vi "Measure.vi"(5 "Progress Ref":refnum<vi>, 7 "XY Graph Reference":refnum<vi>, 8 "error in (no error)":errorcluster, 11 "MCCW ACLR in":refnum<class "MCCW ACLR.lvclass">) -> (0 "error out":errorcluster, 2 "Results":T1[](array[typedef]), 3 "MCCW ACLR out":refnum<class "MCCW ACLR.lvclass">)   [LabVIEW 2020, in "MCCW ACLR.lvclass"]
uses:
  MCCW ACLR.lvclass
  C:/Sandbox/RF Bench/Source Code/WiSpry Test Framework/Measurements/Measurement.lvclass
  XML Handler/Controls/Result Cluster.ctl
  Path Control/Paths.ctl
  MCCW ACLR.lvclass/MCCW ACLR.ctl
  Measurement.lvclass/Measurement.ctl
  Instruments/Spectrum Analyzer/Spectrum Analyzer.lvclass/Spectrum Analyzer.ctl
  Instruments/Vector Signal Generator/Vector Signal Generator.lvclass
  Instruments/Spectrum Analyzer/Spectrum Analyzer.lvclass
  Measurement.lvclass
  Path Control/PathControl.lvclass
  XML Handler/XML Handler.lvclass
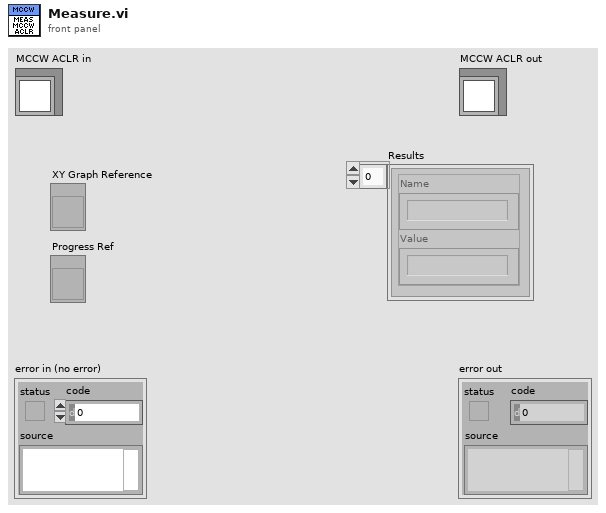
[diagram p1: front panel]
types:
  T1 = typedef "XML Handler.lvclass/Result Cluster.ctl" = cluster{"Name":string, "Value":string}
  T2 = typedef "PathControl.lvclass/Paths.ctl" = enum16{"SigGen 1 -> DUT", "SigGen 2 -> DUT", "SigGen 1 -> PM 1", "SigGen 1 -> PM 2", "DUT -> SA", "DUT -> PM 2", "VSG -> DUT", "SigGen 2 -> PM 1", "SigGen 2 -> PM 2"}
  T3 = cluster{"List":dbl[], "Index":i32, "Last":bool, "BW [MHz]":dbl}
  T4 = cluster{"Number of Measurements":u32, "Current Measurement":u32, "Last":bool}
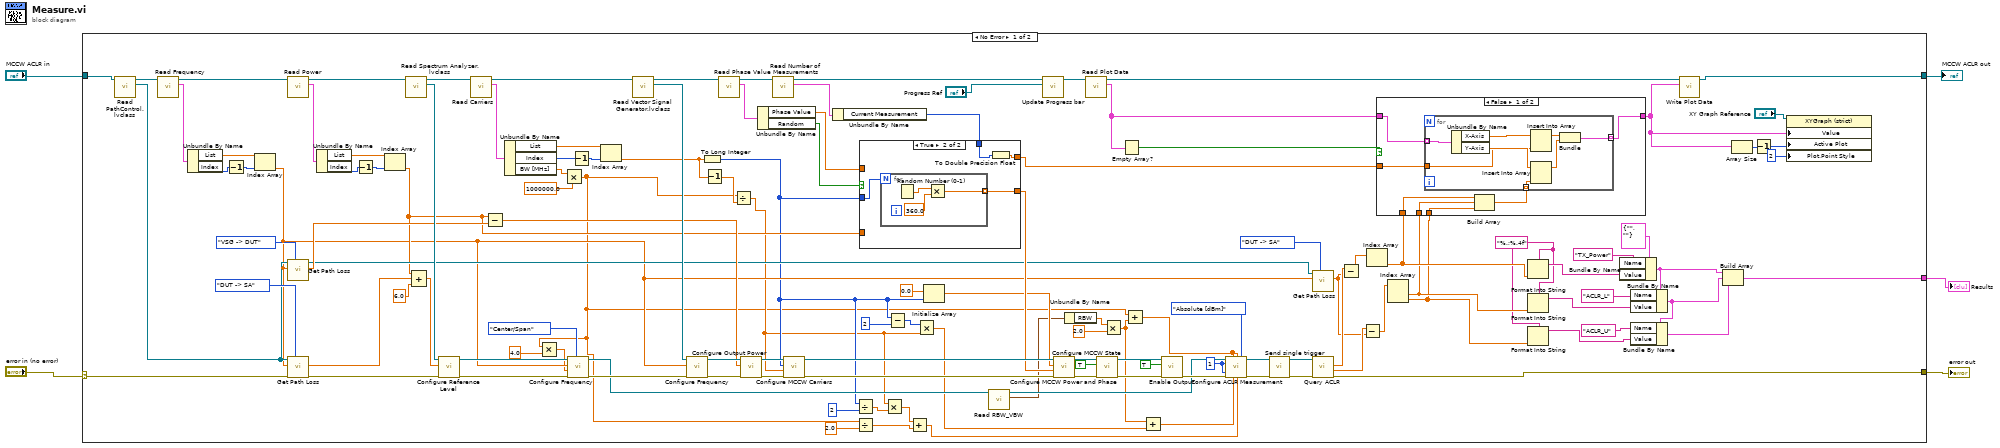
[diagram p0: block diagram]
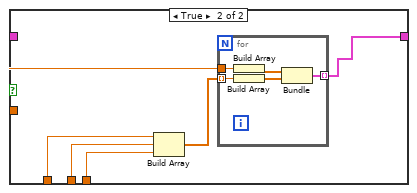
[diagram p2: hidden frame]
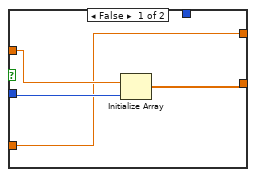
[diagram p3: hidden frame]
diagram:
  n1 = case shown="No Error" "error in (no error)" {
    selector: "error in (no error)" -> [w116 w171]
    tunnel: [w69 w171] -> w4
    tunnel: [w46 w170] -> w2
    tunnel: "MCCW ACLR in" -> [w132 w170]
    tunnel: [w53 _] -> w1
    frame No Error {
      w26 = 1 ("TX Channels")
      w60 = "%.;%.4f" ("format string")
      n2 = call "Read PathControl.lvclass.vi"("Measurements in"=w132) -> ("PathControl.lvclass"=w106:refnum<class "PathControl.lvclass">, "Measurements out"=w131:refnum<class "MCCW ACLR.lvclass">)  [unwired: 9 in]
      n3 = call "Read Frequency.vi"("MCCW ACLR in"=w131) -> ("Frequency"=w126:cluster{"List":dbl[], "Index":i32, "Last":bool}, "MCCW ACLR out"=w130:refnum<class "MCCW ACLR.lvclass">)  [unwired: 9 in]
      n4 = Unbundle By Name(w126) -> ("List"=w129:dbl[], "Index"=w128:i32)
      n5 = Decrement(x=w128) -> (x-1=w127:i32)
      n6 = Index Array(array=w129, index=w127) -> (element=w34:dbl)
      n7 = call "Read Power.vi"("MCCW ACLR in"=w130) -> ("Power"=w122:cluster{"List":dbl[], "Index":i32, "Last":bool}, "MCCW ACLR out"=w115:refnum<class "MCCW ACLR.lvclass">)  [unwired: 9 in]
      n8 = call "Get Path Loss.vi"("Path"=Paths."VSG -> DUT", "Frequency [Hz]"=w34, "PathControl in"=w106) -> ("Insertion Loss (dB)"=w104:dbl, "PathControl out"=w77:refnum<class "PathControl.lvclass">)  [unwired: 5 in, 2 out]
      n9 = call "Get Path Loss.vi"("Path"=Paths."DUT -> SA", "error in (no error)"=w116, "Frequency [Hz]"=w34, "PathControl in"=w106) -> ("error out"=w112:errorcluster, "Insertion Loss (dB)"=w111:dbl)  [unwired: 4 in, 2 out]
      n10 = Unbundle By Name(w122) -> ("List"=w123:dbl[], "Index"=w124:i32)
      n11 = Decrement(x=w124) -> (x-1=w125:i32)
      n12 = Index Array(array=w123, index=w125) -> (element=w68:dbl)
      n13 = call "Read Spectrum Analyzer.lvclass.vi"("MCCW ACLR in"=w115) -> ("Spectrum Analyzer.lvclass"=w113:refnum<class "Spectrum Analyzer.lvclass">, "MCCW ACLR out"=w114:refnum<class "MCCW ACLR.lvclass">)  [unwired: 9 in]
      n14 = Compound Arithmetic op=ADD(w68, w111, 6.0 ("value")) -> (w109:dbl)
      n15 = call-dynamic "Configure Reference Level.vi"("error in (no error)"=w112, "Reference Level [dBm]"=w109, "Spectrum Analyzer in"=w113) -> ("error out"=w35:errorcluster, "Spectrum Analyzer out"=w37:refnum<class "Spectrum Analyzer.lvclass">)  [unwired: 7 in]
      n16 = call "Read Carriers.vi"("MCCW ACLR in"=w114) -> ("Carriers"=w118:T3, "MCCW ACLR out"=w108:refnum<class "MCCW ACLR.lvclass">)  [unwired: 9 in]
      n17 = Subtract(x=w68, y=w104) -> (x-y=w102:dbl)
      n18 = Unbundle By Name(w118) -> ("List"=w121:dbl[], "Index"=w120:i32, "BW [MHz]"=w97:dbl)
      n19 = Multiply(x=w97, y=1000000.0) -> (x*y=w10:dbl)
      n20 = Multiply(x=w10, y=4.0) -> (x*y=w32:dbl)
      n21 = call-dynamic "Configure Frequency.vi"("Mode (Center/Span)"=enum16{"Center/Span", "Start/Stop"}."Center/Span", "error in (no error)"=w35, "Span/Stop Frequency [Hz]"=w32, "Center/Start Frequency [Hz]"=w34, "Spectrum Analyzer in"=w37) -> ("error out"=w36:errorcluster, "Spectrum Analyzer out"=w25:refnum<class "Spectrum Analyzer.lvclass">)  [unwired: 5 in]
      n22 = Decrement(x=w120) -> (x-1=w119:i32)
      n23 = Index Array(array=w121, index=w119) -> (element=w98:dbl)
      n24 = call "Read Vector Signal Generator.lvclass.vi"("MCCW ACLR in"=w108) -> ("Vector Signal Generator.lvclass"=w107:refnum<class "Vector Signal Generator.lvclass">, "MCCW ACLR out"=w92:refnum<class "MCCW ACLR.lvclass">)  [unwired: 9 in]
      n25 = call-dynamic "Configure Frequency.vi"("error in (no error)"=w36, "Frequency [Hz]"=w34, "Signal Generator in"=w107) -> ("error out"=w101:errorcluster, "Signal Generator out"=w103:refnum<class "Vector Signal Generator.lvclass">)  [unwired: 7 in]
      n26 = To Long Integer(number=w98) -> (32bit integer=w14:i32)
      n27 = Decrement(x=w98) -> (x-1=w95:dbl)
      n28 = call "Read Phase Value.vi"("MCCW ACLR in"=w92) -> ("Phase Value"=w91:cluster{"Phase Value":dbl, "Random":bool}, "MCCW ACLR out"=w41:refnum<class "MCCW ACLR.lvclass">)  [unwired: 9 in]
      n29 = Divide(x=w10, y=w95) -> (x/y=w11:dbl)
      n30 = call-dynamic "Configure Output Power.vi"("error in (no error)"=w101, "Output Power [dBm]"=w102, "Signal Generator in"=w103) -> ("error out"=w100:errorcluster, "Signal Generator out"=w99:refnum<class "Vector Signal Generator.lvclass">)  [unwired: 7 in]
      n31 = Unbundle By Name(w91) -> ("Phase Value"=w89:dbl, "Random"=w90:bool)
      n32 = call "Read Number of Measurements.vi"("MCCW ACLR in"=w41) -> ("Number of Measurements"=w39:T4, "MCCW ACLR out"=w40:refnum<class "MCCW ACLR.lvclass">)  [unwired: 9 in]
      n33 = call-dynamic "Configure MCCW Carriers.vi"("error in (no error)"=w100, "MCCW Carrier spacing [Hz]"=w11, "MCCW Carriers"=w14, "Vector Signal Generator in"=w99) -> ("error out"=w94:errorcluster, "Vector Signal Generator out"=w93:refnum<class "Vector Signal Generator.lvclass">)  [unwired: 6 in]
      n34 = Unbundle By Name(w39) -> ("Current Measurement"=w38:u32)
      n35 = Divide(x=w14, y=2) -> (x/y=w12:dbl)
      n36 = Divide(x=w10, y=2.0) -> (x/y=w7:dbl)
      n37 = case shown="True" w90 {
        tunnel: w14 -> [w162 w166]
        tunnel: [w160 w165] -> w88
        tunnel: w89 -> [w161 _]
        tunnel: [w159 w164] -> w71
        tunnel: w68 -> [w159 _]
        tunnel: w38 -> [_ w163]
        frame False {
          n38 = Initialize Array(w161, w162) -> (w160:dbl[])
        }
        frame True {
          n39 = for {
            N: w166 -> [_]
            tunnel: [w167] -> w165 mode=indexing
            n40 = Random Number (0-1)() -> (number: 0 to 1=w169:dbl)
            n41 = Multiply(x=w169, y=360.0) -> (x*y=w167:dbl)
          }
          n42 = To Double Precision Float(number=w163) -> (double precision float=w164:dbl)
        }
      }
      n43 = Multiply(x=w11, y=w12) -> (x*y=w8:dbl)
      n44 = Subtract(x=w14, y=2) -> (x-y=w18:i32)
      n45 = Add(x=w8, y=w7) -> (x+y=w6:dbl)
      n46 = Multiply(x=w18, y=w11) -> (x*y=w17:dbl)
      n47 = Initialize Array(0.0 ("element"), w14) -> (w86:dbl[])
      n48 = call "Read RBW_VBW.vi"("Spectrum Analyzer in"=w25) -> ("RBW/VBW"=w23:cluster{"RBW":dbl, "VBW":dbl}, "Spectrum Analyzer out"=w24:refnum<class "Spectrum Analyzer.lvclass">)  [unwired: 9 in]
      n49 = call "Update Progress bar.vi"("Progress Ref"="Progress Ref", "Measurements In"=w40) -> ("Measurements Out"=w74:refnum<class "MCCW ACLR.lvclass">)  [unwired: 9 in]
      n50 = call-dynamic "Configure MCCW Power and Phase.vi"("error in (no error)"=w94, "Phase"=w88, "Power"=w86, "Vector Signal Generator in"=w93) -> ("error out"=w85:errorcluster, "Vector Signal Generator out"=w84:refnum<class "Vector Signal Generator.lvclass">)  [unwired: 6 in]
      n51 = Unbundle By Name(w23) -> ("RBW"=w22:dbl)
      n52 = call "Read Plot Data.vi"("MCCW ACLR in"=w74) -> ("Plot Data"=w72:cluster{"X-Axis":dbl[], "Y-Axis":dbl[]}[], "MCCW ACLR out"=w52:refnum<class "MCCW ACLR.lvclass">)  [unwired: 9 in]
      n53 = call-dynamic "Configure MCCW State.vi"("error in (no error)"=w85, "State"=TRUE, "Vector Signal Generator in"=w84) -> ("error out"=w82:errorcluster, "Vector Signal Generator out"=w81:refnum<class "Vector Signal Generator.lvclass">)  [unwired: 7 in]
      n54 = Multiply(x=w22, y=2.0) -> (x*y=w15:dbl)
      n55 = Empty Array?(array=w72) -> (empty?=w73:bool)
      n56 = Add(x=w10, y=w15) -> (x+y=w20:dbl)
      n57 = Add(x=w15, y=w17) -> (x+y=w16:dbl)
      n58 = call-dynamic "Enable Output.vi"("error in (no error)"=w82, "Output Enable (F)"=TRUE, "Signal Generator in"=w81) -> ("error out"=w30:errorcluster)  [unwired: 7 in, 1 out]
      n59 = call-dynamic "Configure ACLR Measurement.vi"("Spectrum Analyzer in"=w24, "TX Bandwidth [Hz]"=w20, "TX Spacing [Hz]"=w20, "ALCR Type"=enum16{"Relative [dBc]", "Absolute [dBm]"}."Absolute [dBm]", "TX Channels"=w26, "Adj Channels"=w26, "error in (no error)"=w30, "Adj Bandwidth [Hz]"=w16, "Adj Spacing [Hz]"=w6) -> ("Spectrum Analyzer out"=w29:refnum<class "Spectrum Analyzer.lvclass">, "error out"=w28:errorcluster)  [unwired: 5 in]
      n60 = call-dynamic "Send single trigger.vi"("error in (no error)"=w28, "Spectrum Analyzer in"=w29) -> ("error out"=w79:errorcluster, "Spectrum Analyzer out"=w78:refnum<class "Spectrum Analyzer.lvclass">)  [unwired: 8 in]
      n61 = call "Get Path Loss.vi"("Path"=Paths."DUT -> SA", "Frequency [Hz]"=w34, "PathControl in"=w77) -> ("Insertion Loss (dB)"=w42:dbl)  [unwired: 5 in, 3 out]
      n62 = call-dynamic "Query ACLR.vi"("error in (no error)"=w79, "Spectrum Analyzer in"=w78) -> ("error out"=w69:errorcluster, "ACLR"=w45:dbl[], "Channel Power [dBm]"=w70:dbl[])  [unwired: 6 in, 1 out]
      n63 = Subtract(x=w70, y=w42) -> (x-y=w43:dbl[])
      n64 = Subtract(x=w45, y=w42) -> (x-y=w44:dbl[])
      n65 = Index Array(array=w43) -> (element=w65:dbl)  [unwired: 1 in]
      n66 = Index Array(array=w44) -> (element #1=w63:dbl, element #2=w59:dbl)  [unwired: 2 in]
      n67 = case shown="False" w73 {
        tunnel: w63 -> [w134 w149]
        tunnel: w65 -> [w135 w150]
        tunnel: w72 -> [w139 _]
        tunnel: [w137 w152] -> w47
        tunnel: w59 -> [w133 w148]
        tunnel: w71 -> [w136 w151]
        frame False {
          n68 = Build Array(w135, w134, w133) -> (w138:dbl[])
          n69 = for {
            tunnel: w139 -> [w143] mode=indexing
            tunnel: w138 -> [w142] mode=indexing
            tunnel: [w141] -> w137 mode=indexing
            tunnel: w136 -> [w140]
            n70 = Unbundle By Name(w143) -> ("X-Axis"=w147:dbl[], "Y-Axis"=w146:dbl[])
            n71 = Insert Into Array(array=w147, new element=w140) -> (w145:dbl[])  [unwired: 1 in]
            n72 = Insert Into Array(array=w146, new element=w142) -> (w144:dbl[])  [unwired: 1 in]
            n73 = Bundle("X-Axis"=w145, "Y-Axis"=w144) -> (w141:cluster{"X-Axis":dbl[], "Y-Axis":dbl[]})  [unwired: 1 in]
          }
        }
        frame True {
          n74 = Build Array(w150, w149, w148) -> (w153:dbl[])
          n75 = for {
            tunnel: w151 -> [w158]
            tunnel: w153 -> [w155] mode=indexing
            tunnel: [w154] -> w152 mode=indexing
            n76 = Build Array(w158) -> (w157:dbl[])
            n77 = Build Array(w155) -> (w156:dbl[])
            n78 = Bundle(w157, w156) -> (w154:cluster{dbl[], dbl[]})  [unwired: 1 in]
          }
        }
      }
      n79 = Format Into String(format string=w60, w65) -> (resulting string=w66:string)  [unwired: 2 in, 1 out]
      n80 = Format Into String(format string=w60, w63) -> (resulting string=w62:string)  [unwired: 2 in, 1 out]
      n81 = Format Into String(format string=w60, w59) -> (resulting string=w58:string)  [unwired: 2 in, 1 out]
      n82 = Bundle By Name(cluster=T1 {"Name"="", "Value"=""} ("Result Cluster"), "Name"="TX_Power", "Value"=w66) -> (w57:T1)
      n83 = Bundle By Name(cluster=w57, "Name"="ACLR_L", "Value"=w62) -> (w56:T1)
      n84 = Bundle By Name(cluster=w56, "Name"="ACLR_U", "Value"=w58) -> (w55:T1)
      n85 = call "Write Plot Data.vi"("Plot Data"=w47, "MCCW ACLR in"=w52) -> ("MCCW ACLR out"=w46:refnum<class "MCCW ACLR.lvclass">)  [unwired: 9 in]
      n86 = Build Array(w57, w56, w55) -> (w53:T1[])
      n87 = Array Size(array=w47) -> (size(s)=w51:i32)
      n88 = Decrement(x=w51) -> (x-1=w50:i32)
      n89 = property class="XYGraph (strict)"(reference="XY Graph Reference", "Value"=w47, "Active Plot"=w50, "Plot.Point Style"=u8 2) -> ()  [unwired: 1 in, 2 out]
    }
    frame Error {
    }
  }
  "error out" <- w4
  "MCCW ACLR out" <- w2
  "Results" <- w1
